vi "NI_close.vi"(8 "error in (no error)":errorcluster, 11 "NI cluster in":T2) -> (0 "error out":errorcluster)   [LabVIEW 2016]
uses:
  NI_cluster.ctl
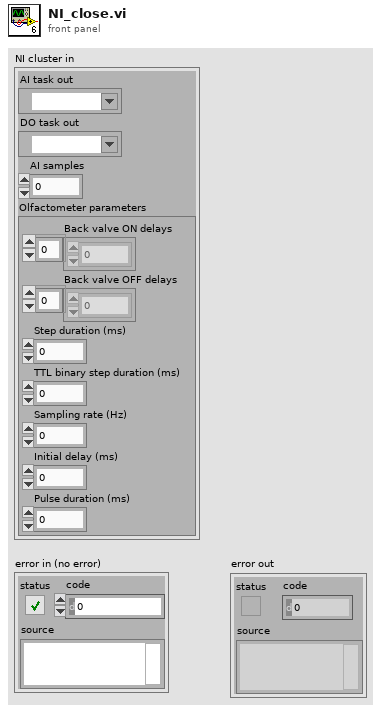
[diagram p1: front panel]
types:
  T1 = typedef "NI_cluster.ctl" = refnum<k21>
  T2 = cluster{"AI task out":refnum<k21>, "DO task out":T1, "AI samples":i32, "Olfactometer parameters":cluster{"Back valve ON delays":dbl[], "Back valve OFF delays":dbl[], "Step duration (ms)":dbl, "TTL binary step duration (ms)":dbl, "Sampling rate (Hz)":dbl, "Initial delay (ms)":dbl, "Pulse duration (ms)":dbl}}
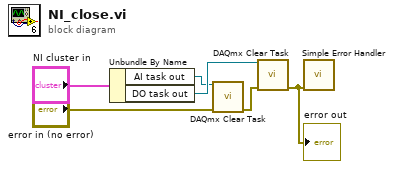
[diagram p0: block diagram]
diagram:
  n1 = Unbundle By Name("NI cluster in") -> ("AI task out"=w5:refnum<k21>, "DO task out"=w6:T1)
  n2 = call <vilib>:"DAQmx Clear Task.vi"("task in"=w5, "error in"="error in (no error)") -> ("error out"=w3:errorcluster)  [unwired: 13 in]
  n3 = call <vilib>:"DAQmx Clear Task.vi"("task in"=w6, "error in"=w3) -> ("error out"=w1:errorcluster)  [unwired: 13 in]
  "error out" <- w1
  n4 = call <vilib>:"Simple Error Handler.vi"("error in (no error)"=w1) -> ()  [unwired: 4 in, 5 out]
